vi "Read JSON File (JSON).vi"(8 "error in (no error)":errorcluster, 11 "file path (use dialog)":path) -> (0 "error out":errorcluster, 3 "Value":T1)   [LabVIEW 2015, in "JSON.lvlib"]
uses:
  JSON.lvlib
  JSON Value.ctl
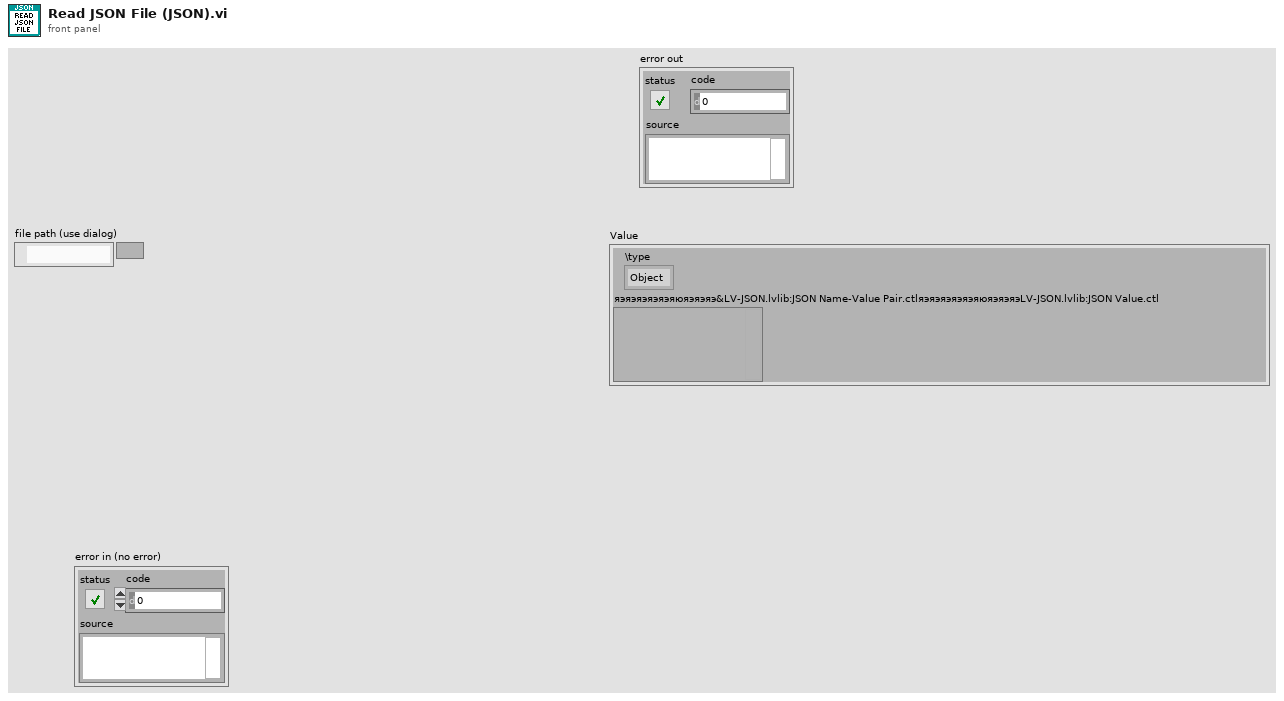
[diagram p1: front panel]
types:
  T1 = typedef "JSON.lvlib/JSON Value.ctl" = cluster{"\\type":enum16{"Object", "Array", "String", "Number", "Boolean", "Null"}, "яэяэяэяэяэяюяэяэяэ&LV-JSON.lvlib:JSON Name-Value Pair.ctlяэяэяэяэяэяюяэяэяэLV-JSON.lvlib:JSON Value.ctl":variant}
  T2 = enum16{"open", "replace", "create", "open or create", "replace or create", "replace or create with confirmation"}
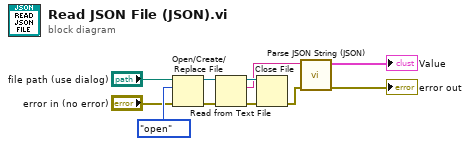
[diagram p0: block diagram]
diagram:
  n1 = Open/Create/Replace File(file path (use dialog)="file path (use dialog)", error in="error in (no error)", operation (0:open)=T2."open") -> (refnum out=w8:refnum<file>, error out=w9:errorcluster)  [unwired: 3 in, 1 out]
  n2 = Read from Text File(file (use dialog)=w8, error in=w9) -> (refnum out=w6:refnum<file>, text=w4:string, error out=w7:errorcluster)  [unwired: 2 in, 1 out]
  n3 = Close File(refnum=w6, error in=w7) -> (error out=w3:errorcluster)  [unwired: 1 out]
  n4 = call "Parse JSON String (JSON).vi"("error in (no error)"=w3, "String"=w4) -> ("error out"=→"error out":errorcluster, "Value"=→"Value":T1)  [unwired: 8 in]
